vi "BuildCall.vi"(7 "PythonConverter_BD in":refnum<class "PyConvBD.lvclass">, 8 "error in":errorcluster, 11 "Local in":refnum<class "Local.lvclass">) -> (0 "error out":errorcluster, 3 "Local out":refnum<class "Local.lvclass">, 5 "PythonConverter_BD out":refnum<class "PyConvBD.lvclass">)   [LabVIEW 2014, in "Raspberry Pi Compatible Compiler for LabVIEW.lvlib" / "Local.lvclass"]
uses:
  Local.lvclass
  Python/PythonConverter_BD/PyConvBD.lvclass
  Python/PythonConverter_BD/TypeDefs/NodeCall_TD.ctl
  Python/Parsing/ListTypesTD.ctl
  Terminal/Terminal.lvclass
  Python/Parsing/Python Functions.lvlib
  Raspberry Pi Compatible Compiler for LabVIEW.lvlib
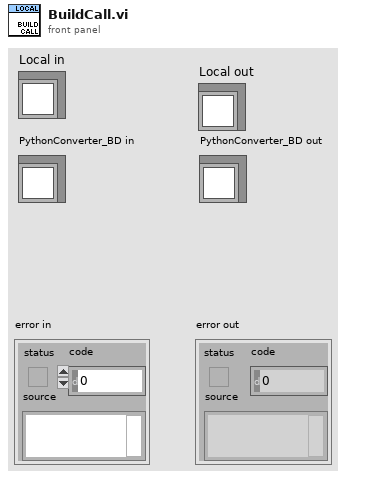
[diagram p1: front panel]
types:
  T1 = typedef "Raspberry Pi Compatible Compiler for LabVIEW.lvlib/NodeCall_TD.ctl" = cluster{"call":string, "collect":string, "Threaded":bool, "branches":string[]}
  T2 = typedef "Raspberry Pi Compatible Compiler for LabVIEW.lvlib/Python Functions.lvlib/ListTypesTD.ctl" = enum16{"list", "tuple", "parameter list", "output list", "return values"}
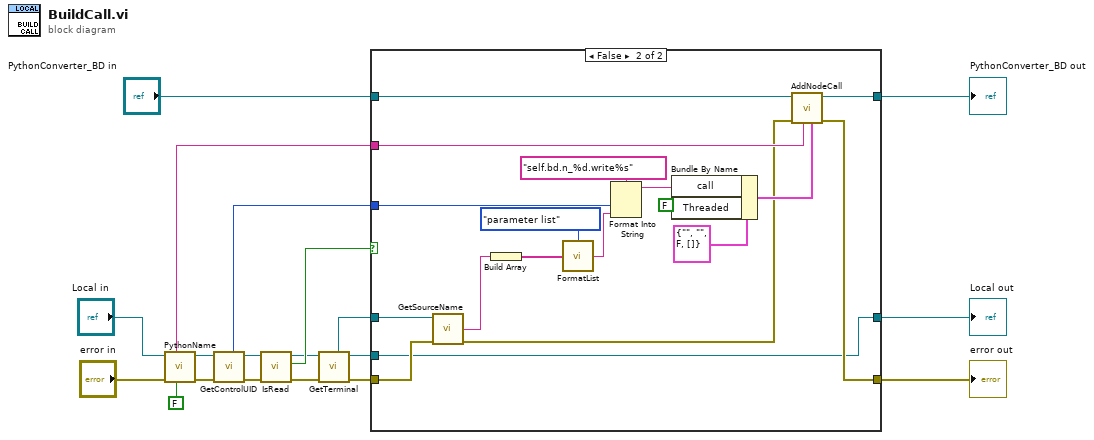
[diagram p0: block diagram]
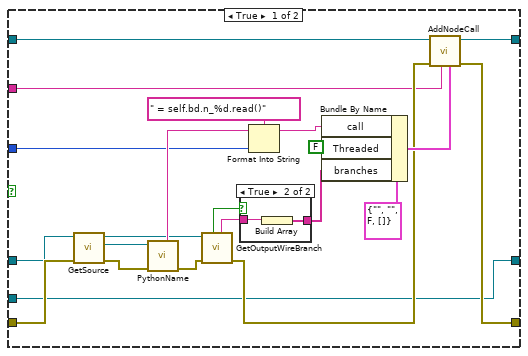
[diagram p2: hidden frame]
diagram:
  n1 = call-dynamic "PythonName.vi"("add self"=FALSE, "error in"="error in", "Node in"="Local in") -> ("error out"=w4:errorcluster, "Node out"=w5:refnum<class "Local.lvclass">, "UID"=w11:string)  [unwired: 5 in, 1 out]
  n2 = call "GetControlUID.vi"("error in"=w4, "Local in"=w5) -> ("error out"=w2:errorcluster, "Local out"=w3:refnum<class "Local.lvclass">, "UID"=w1:i32)  [unwired: 5 in]
  n3 = call-dynamic "IsRead.vi"("error in"=w2, "Local in"=w3) -> ("error out"=w9:errorcluster, "is read"=w13:bool, "Local out"=w10:refnum<class "Local.lvclass">)  [unwired: 5 in]
  n4 = call "GetTerminal.vi"("error in"=w9, "Local in"=w10) -> ("error out"=w8:errorcluster, "Local out"=w6:refnum<class "Local.lvclass">, "terminal"=w7:refnum<class "Terminal.lvclass">)  [unwired: 5 in]
  n5 = case shown="False" w13 {
    tunnel: w7 -> [w40 w47]
    tunnel: w8 -> [w41 w46]
    tunnel: "PythonConverter_BD in" -> [w36 w57]
    tunnel: [w35 w56] -> w17
    tunnel: [w34 w55] -> w18
    tunnel: [w22 w45] -> w16
    tunnel: w11 -> [w20 w54]
    tunnel: w6 -> [w22 w45]
    tunnel: w1 -> [w21 w44]
    frame True {
      n6 = call "GetSource.vi"("error in"=w41, "Terminal in"=w40) -> ("error out"=w39:errorcluster, "source"=w38:refnum<class "Terminal.lvclass">, "Terminal out"=w28:refnum<class "Terminal.lvclass">)  [unwired: 5 in]
      n7 = call-dynamic "PythonName.vi"("error in"=w39, "Terminal in"=w38) -> ("error out"=w27:errorcluster, "name"=w33:string)  [unwired: 6 in, 2 out]
      n8 = call-dynamic "GetOutputWireBranch.vi"("error in"=w27, "Terminal in"=w28) -> ("error out"=w26:errorcluster, "branches"=w24:string, "branched"=w25:bool)  [unwired: 4 in, 1 out]
      n9 = case shown="True" w25 {
        tunnel: w24 -> [_ w43]
        tunnel: [_ w42] -> w23
        frame False {
        }
        frame True {
          n10 = Build Array(w43) -> (w42:string[])
        }
      }
      n11 = Format Into String(format string=" = self.bd.n_%d.read()", initial string=w33, w21) -> (resulting string=w29:string)  [unwired: 1 in, 1 out]
      n12 = Bundle By Name(cluster=T1 {"call"="", "collect"="", "Threaded"=FALSE, "branches"=[]} ("call"), "call"=w29, "Threaded"=FALSE, "branches"=w23) -> (w30:T1)
      n13 = call "AddNodeCall.vi"("call"=w30, "name"=w20, "error in"=w26, "PythonConverter_BD in"=w36) -> ("error out"=w35:errorcluster, "PythonConverter_BD out"=w34:refnum<class "PyConvBD.lvclass">)  [unwired: 4 in]
    }
    frame False {
      n14 = call "GetSourceName.vi"("error in"=w46, "Terminal in"=w47) -> ("error out"=w49:errorcluster, "source"=w48:string)  [unwired: 5 in, 1 out]
      n15 = Build Array(w48) -> (w58:string[])
      n16 = call "FormatList.vi"("values"=w58, "type"=ListTypesTD."parameter list") -> ("python object"=w59:string)
      n17 = Format Into String(format string="self.bd.n_%d.write%s", w44, w59) -> (resulting string=w51:string)  [unwired: 2 in, 1 out]
      n18 = Bundle By Name(cluster=T1 {"call"="", "collect"="", "Threaded"=FALSE, "branches"=[]} ("call"), "call"=w51, "Threaded"=FALSE) -> (w50:T1)
      n19 = call "AddNodeCall.vi"("call"=w50, "name"=w54, "error in"=w49, "PythonConverter_BD in"=w57) -> ("error out"=w56:errorcluster, "PythonConverter_BD out"=w55:refnum<class "PyConvBD.lvclass">)  [unwired: 4 in]
    }
  }
  "error out" <- w17
  "Local out" <- w16
  "PythonConverter_BD out" <- w18
